vi "boolean_to_string.vi"(8 "error in (no error)":errorcluster, 10 "Boolean":bool=TRUE) -> (0 "error out":errorcluster, 2 "String":string)   [LabVIEW 2018]
doc: "Format a float as an IC6 defined REAL_4X1 string."
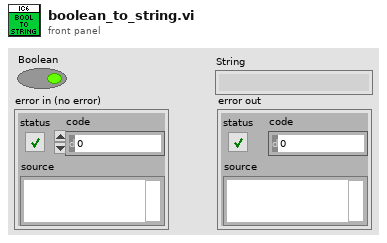
[diagram p1: front panel]
types:
  T1 = enum16{"big-endian, network order", "native, host order", "little-endian"}
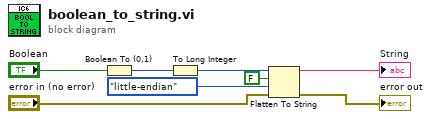
[diagram p0: block diagram]
diagram:
  n1 = Boolean To (0,1)(Boolean="Boolean") -> (0, 1=w6:i16)
  n2 = To Long Integer(number=w6) -> (32bit integer=w5:i32)
  n3 = Flatten To String(anything=w5, prepend array or string size? (T)=FALSE, byte order (0:big-endian, network order)=T1."little-endian", error in (no error)="error in (no error)") -> (data string=→"String":string, error out=→"error out":errorcluster)  [unwired: 1 out]
